vi "MenuPruebas.vi"(8 "error in (no error)":errorcluster, 11 "Equipo.lvclass":refnum<class "Equipo.lvclass">) -> (0 "error out":errorcluster)   [LabVIEW 2019, in "Aplicacion.lvclass"]
uses:
  Aplicacion.lvclass
  Equipo/Equipo/Equipo.lvclass
  Pruebas/Prueba/Prueba.lvclass/Prueba.ctl
  <vilib>/Utility/error.llb/Trim Whitespace.vi
  Pruebas/Prueba/Prueba.lvclass
panel:
  in  "condi_ambient_finales":bool
  in  "Certificado":bool
  out "estadoPruebas":i32(listbox)
  in  "ir_a_prueba":bool
  in  "listaPruebas":i32(listbox)
  in  "Salir":bool
  # "MENU DE PRUEBAS"
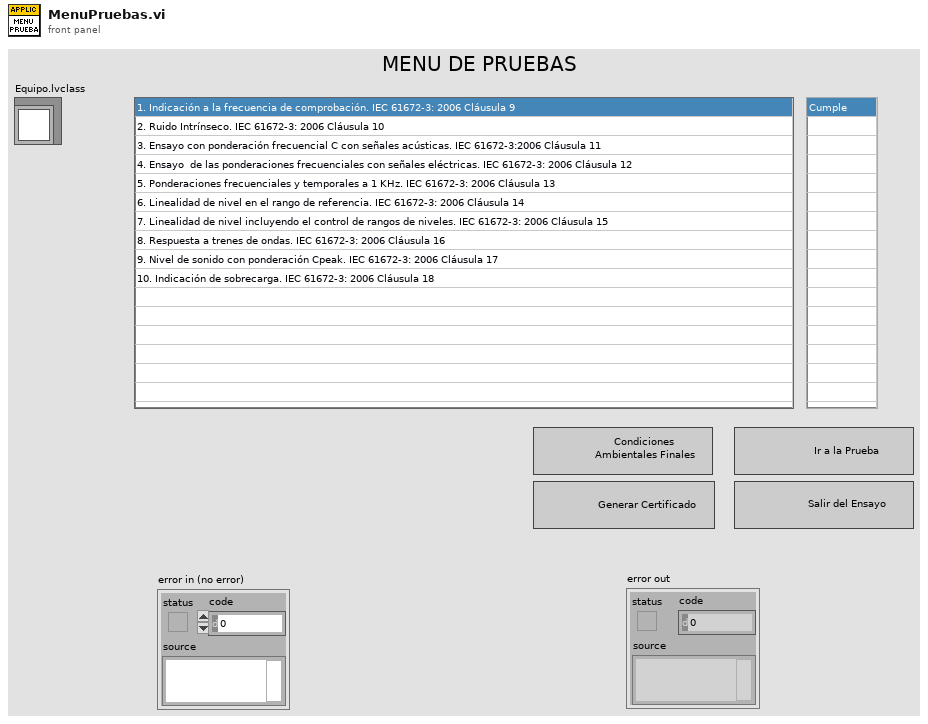
[diagram p1: front panel]
types:
  T1 = enum8{"Enabled", "Disabled", "Disabled and Grayed Out"}
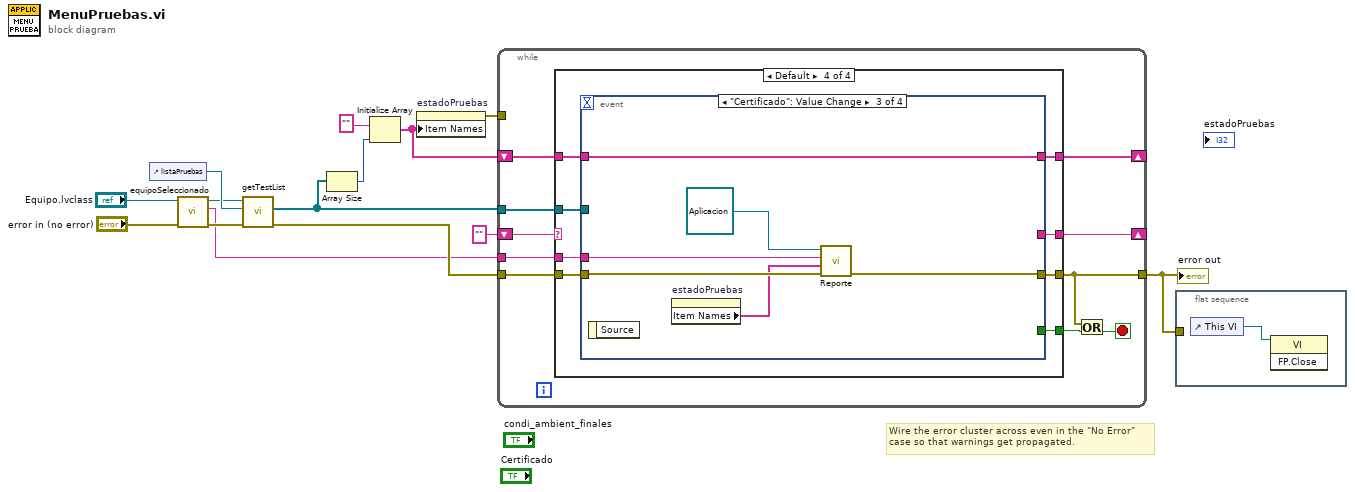
[diagram p0: block diagram]
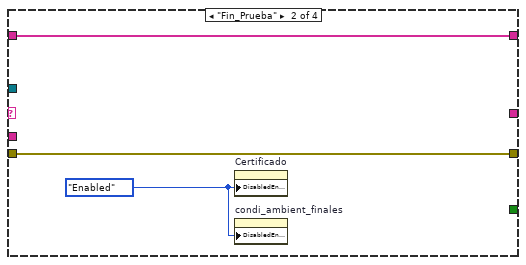
[diagram p3: hidden frame]
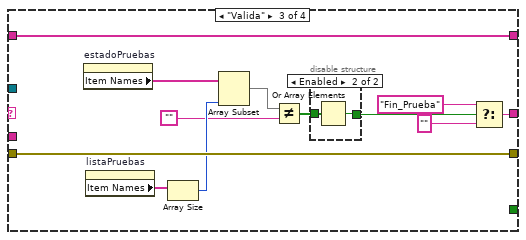
[diagram p4: hidden frame]
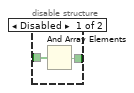
[diagram p5: hidden frame]
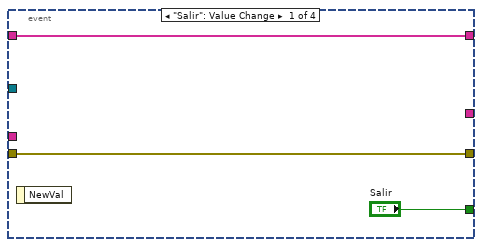
[diagram p6: hidden frame]
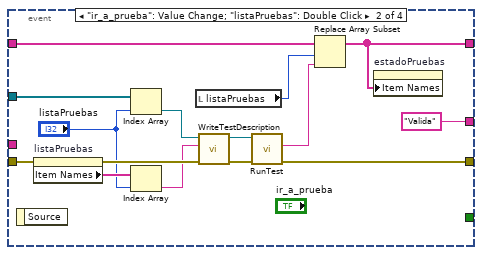
[diagram p7: hidden frame]
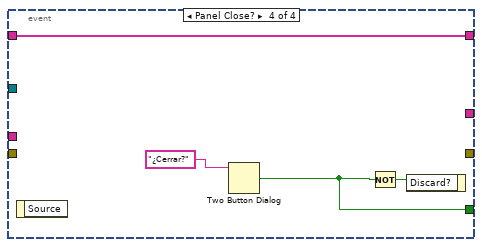
[diagram p8: hidden frame]
diagram:
  # "Wire the error cluster across even in the \"No Error\"\ncase so that warnings get propagated."
  n1 = control-ref of="listaPruebas"() -> (w14:refnum<vi>)
  n2 = call-dynamic "equipoSeleccionado.vi"("error in (no error)"="error in (no error)", "Equipo in"="Equipo.lvclass") -> ("error out"=w2:errorcluster, "equipoSeleccionado"=w1:string, "Equipo out"=w3:refnum<class "Equipo.lvclass">)  [unwired: 7 in]
  n3 = call-dynamic "getTestList.vi"("error in (no error)"=w2, "listaPruebas"=w14, "Equipo in"=w3) -> ("error out"=w13:errorcluster, "listaDePruebas"=w7:refnum<class "Prueba.lvclass">[])  [unwired: 6 in, 1 out]
  n4 = Array Size(array=w7) -> (size(s)=w8:i32)
  n5 = Initialize Array("", w8) -> (w6:string[])
  n6 = property on="estadoPruebas" class="LstBox (strict)"("Item Names"=w6) -> (error out=w11:errorcluster)  [unwired: 2 in, 1 out]
  n7 = while {
    tunnel: w7 -> [w23]
    tunnel: w13 -> [w22]
    tunnel: [w20] -> w12
    tunnel: w11 -> [_]
    shift-right: [w18] -> _
    shift-left: w6 -> [w19]
    shift-right: [w16] -> _
    shift-left: "" -> [w17]
    tunnel: w1 -> [w15]
    stop <- w21 stop-if-true
    n8 = case shown="Default" w17 {
      tunnel: [_ _ _ w53] -> w24
      tunnel: w23 -> [_ _ _ w52]
      tunnel: w22 -> [w26 w28 w40 w51]
      tunnel: [w26 w28 w40 w50] -> w20
      tunnel: w19 -> [w25 w29 w41 w49]
      tunnel: [w25 w29 w41 w48] -> w18
      tunnel: [_ _ w30 w47] -> w16
      tunnel: w15 -> [_ _ _ w46]
      frame "Certificado" {
      }
      frame "Fin_Prueba" {
        w27 = T1."Enabled" ("Disabled")
        n9 = property on="Certificado" class="Bool"("DisabledEnum"=w27) -> ()  [unwired: 2 in, 2 out]
        n10 = property on="condi_ambient_finales" class="Bool"("DisabledEnum"=w27) -> ()  [unwired: 2 in, 2 out]
      }
      frame "Valida" {
        n11 = property on="estadoPruebas" class="LstBox (strict)"() -> ("Item Names"=w38:string[])  [unwired: 2 in, 2 out]
        n12 = property on="listaPruebas" class="LstBox (strict)"() -> ("Item Names"=w39:string[])  [unwired: 2 in, 2 out]
        n13 = Array Size(array=w39) -> (size(s)=w37:i32)
        n14 = Array Subset(array=w38, length=w37) -> (w36:string[])  [unwired: 1 in]
        n15 = Not Equal?(x=w36, y="") -> (x != y?=w34:bool[])
        n16 = disable-structure shown="Enabled" {
          disable-tunnel: w34 -> [w43 w45]
          disable-tunnel: [w42 w44] -> w33
          frame Disabled {
            n17 = And Array Elements(Boolean array=w43) -> (logical AND=w42:bool)
          }
          frame Enabled {
            n18 = Or Array Elements(Boolean array=w45) -> (logical OR=w44:bool)
          }
        }
        n19 = Select(t="Fin_Prueba", s=w33, f="") -> (s? t:f=w30:string)
      }
      frame Default {
        n20 = event shown="[2] \"Certificado\": Value Change" {
          selector: _ -> [_ _ _ _]
          dyn-events: _ -> [_ _ _ _]
          timeout: _ -> [_ _ _ _]
          tunnel: ["Salir" _ _ w78] -> w53
          tunnel: w52 -> [_ w71 _ _]
          tunnel: w51 -> [w55 w62 w76 _]
          tunnel: [w55 w70 w75 _] -> w50
          tunnel: w49 -> [w54 w67 w77 w79]
          tunnel: [w54 w66 w77 w79] -> w48
          tunnel: [_ "Valida" _ _] -> w47
          tunnel: w46 -> [_ _ w73 _]
          event "Salir": Value Change {
            n21 = event-data() -> ()  [unwired: 1 in, 1 out]
          }
          event "ir_a_prueba": Value Change; "listaPruebas": Double Click {
            n22 = event-data() -> ()  [unwired: 1 in, 1 out]
            n23 = property on="listaPruebas" class="LstBox (strict)"(error in=w62) -> (error out=w61:errorcluster, "Item Names"=w60:string[])  [unwired: 1 in, 1 out]
            n24 = Index Array(array=w71, index="listaPruebas") -> (element=w65:refnum<class "Prueba.lvclass">)
            n25 = Index Array(array=w60, index="listaPruebas") -> (element=w58:string)
            n26 = local read "listaPruebas"() -> (w69:i32)
            n27 = call "WriteTestDescription.vi"("error in (no error)"=w61, "Test Description"=w58, "Prueba in"=w65) -> ("error out"=w63:errorcluster, "Prueba out"=w64:refnum<class "Prueba.lvclass">)  [unwired: 7 in]
            n28 = call-dynamic "RunTest.vi"("error in (no error)"=w63, "Prueba in"=w64) -> ("error out"=w70:errorcluster, "resultado"=w68:string)  [unwired: 7 in, 1 out]
            n29 = Replace Array Subset(array=w67, new element=w68, index=w69) -> (w66:string[])
            n30 = property on="estadoPruebas" class="LstBox (strict)"("Item Names"=w66) -> ()  [unwired: 2 in, 2 out]
          }
          event "Certificado": Value Change {
            n31 = event-data() -> ()  [unwired: 1 in, 1 out]
            n32 = property on="estadoPruebas" class="LstBox (strict)"() -> ("Item Names"=w72:string[])  [unwired: 2 in, 2 out]
            n33 = call "Reporte.vi"("error in (no error)"=w76, "Estado"=w72, "Equipo"=w73, "Aplicacion in"=refnum<class "Aplicacion.lvclass"> refnum) -> ("error out"=w75:errorcluster)  [unwired: 6 in, 1 out]
          }
          event Panel Close? {
            n34 = event-data() -> ()  [unwired: 1 in, 1 out]
            n35 = Two Button Dialog(message="¿Cerrar?") -> (T button?=w78:bool)  [unwired: 2 in]
            n36 = Not(x=w78) -> (.not. x?=w80:bool)
            n37 = event-data("Discard?"=w80) -> ()  [unwired: 1 in, 1 out]
          }
        }
      }
    }
    n38 = Or(x=w20, y=w24) -> (x .or. y?=w21:bool)
  }
  "error out" <- w12
  n39 = flat-sequence {
    tunnel: w12 -> [_]
    frame #0 {
      n40 = control-ref of="This VI"() -> (w82:refnum<vi>)
      n41 = invoke class="VI" method="FP.Close"(reference=w82) -> ()  [unwired: 2 in, 3 out]
    }
  }
